vi "CTRE_PigeonIMU_Open_CAN.vi"(8 "error in":errorcluster, 10 "Device Number":u8) -> (0 "error out":errorcluster, 3 "PigeonIMUDevRef":T1={"DeviceStatus"={"status"=FALSE, "code"=0, "source"=""}, "Device Number"=0, "Type"=352321536, "Device ID"=0} {"Type" items=["CAN"=352321536, "TalonSRX"=33554432]})   [LabVIEW 2016]
doc: "Opens a Pigeon IMU Device Reference using a CAN ID."
uses:
  <vilib>/Rock Robotics/WPI/ThirdParty/Sensors/Pigeon IMU/CTRE_PigeonIMU_DeviceRef.ctl
  <vilib>/Rock Robotics/WPI/ThirdParty/Sensors/Pigeon IMU/CTRE_PigeonIMU_ConnectionType.ctl
  <vilib>/Rock Robotics/WPI/ThirdParty/Sensors/Pigeon IMU/CTRE_PigeonIMU_MessageIDs.ctl
  <vilib>/Rock Robotics/WPI/ThirdParty/Sensors/Pigeon IMU/CTRE_PigeonIMU_UsageTypes.ctl
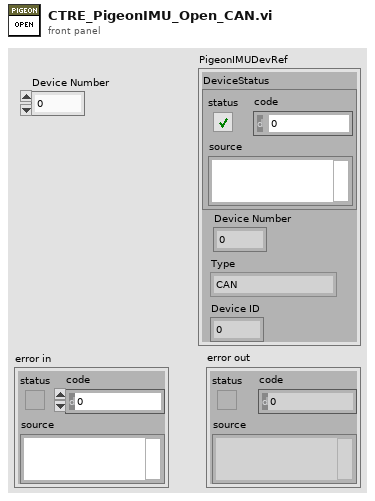
[diagram p1: front panel]
types:
  T1 = typedef "CTRE_PigeonIMU_DeviceRef.ctl" = cluster{"DeviceStatus":errorcluster, "Device Number":u8, "Type":T2, "Device ID":u32}
  T2 = typedef "CTRE_PigeonIMU_ConnectionType.ctl" = u32
  T3 = typedef "CTRE_PigeonIMU_UsageTypes.ctl" = u32
  T4 = typedef "CTRE_PigeonIMU_MessageIDs.ctl" = u32
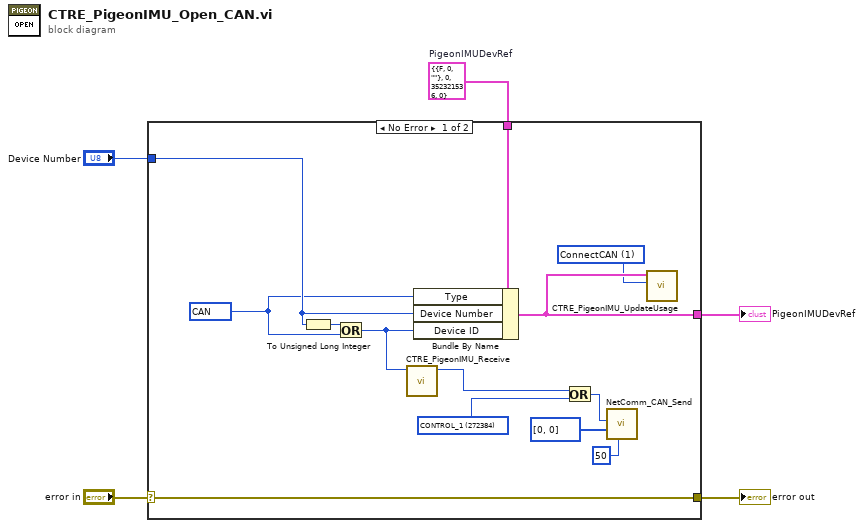
[diagram p0: block diagram]
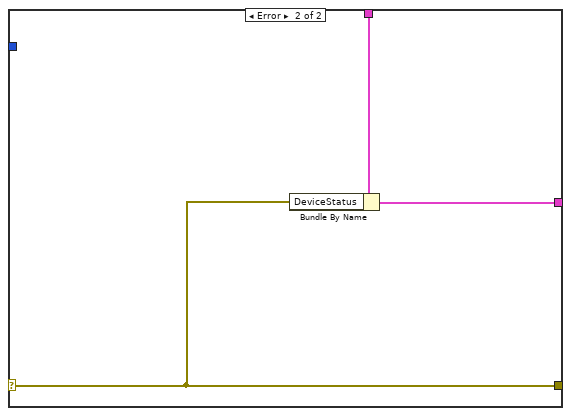
[diagram p2: hidden frame]
diagram:
  w3 = T1 {"DeviceStatus"={"status"=FALSE, "code"=0, "source"=""}, "Device Number"=0, "Type"=352321536, "Device ID"=0}  # PigeonIMUDevRef
  n1 = case shown="No Error" "error in" {
    selector: "error in" -> [w18 w20]
    tunnel: [w18 w20] -> w4
    tunnel: w3 -> [w17 w21]
    tunnel: [w7 w19] -> w2
    tunnel: "Device Number" -> [w15 _]
    frame No Error {
      w6 = T3 1 items=["Defaul"=0, "ConnectCAN"=1, "ConnectTalonSRX"=2, "GetCompass"=134217728, "GetYPR"=268435456, "GetFused"=536870912, "GetAccel"=1073741824, "TempComp"=2147483648] ("Usage")
      w8 = T2 352321536 items=["CAN"=352321536, "TalonSRX"=33554432] ("Connection Type")
      w14 = T4 272384 items=["RAW_STATUS_2"=265280, "RAW_STATUS_4"=265408, "RAW_STATUS_6"=265536, "BIASED_STATUS_2"=269376, "BIASED_STATUS_4"=269504, "BIASED_STATUS_6"=269632, "COND_STATUS_1"=270336, "COND_STATUS_2"=270400, "COND_STATUS_3"=270464, "COND_STATUS_4"=270528, "COND_STATUS_5"=270592, "COND_STATUS_6"=270656, "COND_STATUS_7"=270720, "COND_STATUS_8"=270784, "COND_STATUS_9"=270848, "COND_STATUS_10"=270912, "CONTROL_1"=272384, "PARAM_REQUEST"=273408, "PARAM_RESPONSE"=273472, "PARAM_SET"=273536] ("MessageIDs")
      n2 = To Unsigned Long Integer(number=w15) -> (unsigned 32bit integer=w16:u32)
      n3 = Or(x=w16, y=w8) -> (x .or. y?=w10:T2)
      n4 = call <vilib>:"CTRE_PigeonIMU_Receive.vi"("Device ID"=w10) -> ("Device ID Out"=w9:u32)  [unwired: 10 in]
      n5 = Bundle By Name(cluster=w17, "Type"=w8, "Device Number"=w15, "Device ID"=w10) -> (w7:T1)
      n6 = Or(x=w9, y=w14) -> (x .or. y?=w13:T4)
      n7 = call <vilib>:"NetComm_CAN_Send.vi"("Period (ms)"=50, "Data"=u8[] [0, 0], "Message ID"=w13) -> ()  [unwired: 8 in, 1 out]
      n8 = call <vilib>:"CTRE_PigeonIMU_UpdateUsage.vi"("Usage"=w6, "PigeonIMUDevRef"=w7) -> ()  [unwired: 10 in]
    }
    frame Error {
      n9 = Bundle By Name(cluster=w21, "DeviceStatus"=w20) -> (w19:T1)
    }
  }
  "error out" <- w4
  "PigeonIMUDevRef" <- w2
